vi "BCU诊断标定.vi"(8 "CAN端口":u16(ring), 9 "设备索引号":u16(ring), 10 "CAN卡类型":u32(ring)=21, 11 "Myindex":dbl=1.0) -> (3 "成功":bool)   [LabVIEW 2013] (continued)
                    n2819 = Enqueue Element(queue=w3690, element="强制均衡" ("元素"), error in (no error)=w3689) -> (queue out=w3687:refnum<queue>, error out=w3686:errorcluster)  [unwired: 2 out]
                  }
                }
                n2820 = call <vilib>:"Set Busy.vi"("disable click? (T)"=TRUE) -> ()  [unwired: 3 in, 8 out]
              }
            }
          }
        }
        n2821 = Unbundle By Name(w901) -> ("status"=w900:bool)
        n2822 = Or(x=w900, y=w902) -> (x .or. y?=w903:bool)
      }
      n2823 = Release Queue(queue=w896, force destroy? (F)=TRUE ("强制销毁？(F)"), error in (no error)=w895) -> (error out=w893:errorcluster)  [unwired: 2 out]
      n2824 = call <vilib>:"Clear Errors.vi"("error in (no error)"=w893) -> ()  [unwired: 7 out]
    }
    frame Disabled {
    }
  }
  n2825 = while {
    tunnel: w39 -> [w3702]
    tunnel: w38 -> [w3701]
    tunnel: [w3700] -> w42
    tunnel: [w3699] -> w41
    tunnel: w34 -> [_]
    tunnel: w37 -> [w3691]
    stop <- w3698 stop-if-true
    n2826 = local read "停止"() -> (w3698:bool)
    n2827 = local read "设备索引号"() -> (w3695:u16)
    n2828 = local read "CAN卡类型"() -> (w3696:u32)
    n2829 = local read "CAN端口"() -> (w3694:u16)
    n2830 = call "receiver-8.6.vi"("错误输入（无错误）"=w3691, "CAN端口"=w3694, "设备索引号"=w3695, "CAN卡类型"=w3696) -> ("错误输出"=w3697:errorcluster, "输出簇"=w3693:T25, "接收成功"=w3692:bool)  [unwired: 3 out]
    n2831 = call <vilib>:"Clear Errors.vi"("error in (no error)"=w3697) -> ()  [unwired: 6 in, 1 out]
    n2832 = case shown="真" w3692 {
      tunnel: w3701 -> [w3703 w3709]
      tunnel: w3693 -> [_ w3708]
      tunnel: w3702 -> [w3704 w3707]
      tunnel: [w3704 w3706] -> w3700
      tunnel: [w3703 w3705] -> w3699
      frame False {
      }
      frame True {
        n2833 = Enqueue Element(queue=w3707, element=w3708, error in (no error)=w3709) -> (queue out=w3706:refnum<queue>, error out=w3705:errorcluster)  [unwired: 2 out]
      }
    }
  }
  n2834 = while {
    tunnel: w39 -> [w3717]
    tunnel: w38 -> [w3716]
    stop <- w3710 stop-if-true
    n2835 = local read "停止"() -> (w3710:bool)
    n2836 = local read "控制1"() -> (w3712:bool)
    n2837 = Dequeue Element(queue=w3717, timeout in ms (-1)=200 ("超时毫秒(-1)"), error in (no error)=w3716) -> (element=w3715:T3, error out=w3714:errorcluster)  [unwired: 2 out]
    n2838 = case shown="无错误" w3714 {
      tunnel: w3715 -> [w3722 _]
      tunnel: "写?" -> [w3719 _]
      tunnel: w3712 -> [w3718 _]
      frame No Error {
        n2839 = Unbundle(w3722) -> ("return type"=w3721:u32, "pReceive"=w3720:T26)
        n2840 = for {
          N: w3721 -> [_]
          tunnel: w3720 -> [w3726] mode=indexing
          tunnel: w3719 -> [w3724]
          tunnel: w3718 -> [w3723]
          n2841 = Unbundle By Name(w3726) -> ("ID"=w3727:u32)
          n2842 = call "ID解析.vi"("ID"=w3727) -> ("PDU(1)"=w3725:i32)  [unwired: 10 out]
          n2843 = case shown="18" w3725 {
            tunnel: w3726 -> [_ w3737]
            tunnel: w3724 -> [_ w3729]
            tunnel: w3723 -> [_ w3728]
            frame 0, Default {
            }
            frame 24 {
              n2844 = local read "主从选择"() -> (w3730:enum32{"主板", "从板"})
              n2845 = local read "设备索引号"() -> (w3733:u16)
              n2846 = local read "CAN卡类型"() -> (w3732:u32)
              n2847 = local read "CAN端口"() -> (w3734:u16)
              n2848 = disable-structure shown="禁用" {
                disable-tunnel: w3737 -> [w3740 _]
                frame Disabled {
                  n2849 = call "标定授权读取.vi"("VCI_Receive"=w3740) -> ()  [unwired: 1 out]
                }
                frame Enabled {
                }
              }
              n2850 = case shown="\"从板\"" w3730 {
                tunnel: [0 ("FUNC") w3739] -> w3731
                frame "主板", Default {
                }
                frame "从板" {
                  n2851 = local read "从板号"() -> (w3739:u8)
                }
              }
              n2852 = local read "面板选择"() -> (w3736:T7)
              n2853 = case shown="\"读写参数\", 默认" w3736 {
                tunnel: w3729 -> [w3747 _ _ _]
                tunnel: "命令" -> [w3748 w3848 w4103 w4243]
                tunnel: w3730 -> [w3757 _ w4111 w4251]
                tunnel: w3737 -> [_ _ _ _]
                tunnel: w3737 -> [w3753 w3849 w4105 w4245]
                tunnel: w3734 -> [w3752 w3850 w4106 w4246]
                tunnel: w3733 -> [w3751 w3851 w4107 w4247]
                tunnel: w3732 -> [w3750 w3852 w4108 w4248]
                tunnel: w3731 -> [w3749 _ w4104 w4244]
                tunnel: w3728 -> [w3743 _ _ _]
                frame "读写参数", Default {
                  n2854 = control-ref of="流控帧 2"() -> (w3741:refnum<vi>)
                  n2855 = control-ref of="流控帧"() -> (w3742:refnum<vi>)
                  n2856 = local read "命令序号"() -> (w3746:u8)
                  n2857 = call "多帧接收机制(EV05).vi"("can卡类型"=w3750, "设备索引号"=w3751, "CAN端口"=w3752, "VCI_Receive"=w3753, "命令"=w3748, "板号"=w3749, "流控帧"=w3742, "写?"=w3747, "流控帧2"=w3741, "命令序号"=w3746) -> ("错误信号"=w3744:bool, "错误代码"=w3756:i32, "输出数组"=w3755:u8[], "读错误代码"=w3745:u8[], "结束信号"=w3754:bool)  [unwired: 5 out]
                  n2858 = case shown="真" w3747 {
                    tunnel: w3754 -> [w3767 w3830]
                    tunnel: w3756 -> [w3766 w3829]
                    tunnel: w3746 -> [w3765 _]
                    tunnel: w3755 -> [w3764 _]
                    tunnel: w3748 -> [w3763 _]
                    tunnel: w3757 -> [w3761 w3828]
                    tunnel: w3745 -> [w3760 _]
                    tunnel: w3744 -> [w3759 _]
                    tunnel: w3743 -> [w3758 _]
                    frame False {
                      # "读参数"
                      n2859 = And(x=w3758, y=w3767) -> (x .and. y?=w3762:bool)
                      n2860 = case shown="真" w3762 {
                        tunnel: w3766 -> [_ w3778]
                        tunnel: w3765 -> [_ w3777]
                        tunnel: w3764 -> [_ w3776]
                        tunnel: w3763 -> [_ w3775]
                        tunnel: w3761 -> [_ w3771]
                        tunnel: w3760 -> [_ w3769]
                        tunnel: w3759 -> [_ w3770]
                        frame False {
                        }
                        frame True {
                          n2861 = case shown="假" w3770 {
                            tunnel: w3778 -> [w3787 _]
                            tunnel: w3777 -> [w3786 _]
                            tunnel: w3776 -> [w3785 _]
                            tunnel: w3775 -> [w3783 _]
                            tunnel: w3771 -> [w3779 _]
                            tunnel: w3769 -> [_ w3813]
                            frame False {
                              n2862 = case shown="\"主板\", 默认" w3779 {
                                tunnel: [w3788 _] -> w3782
                                tunnel: [_ w3801] -> w3781
                                frame "主板", Default {
                                n2863 = stacked-sequence {
                                tunnel: [_ w3800] -> w3788
                                frame #0 {
                                n2864 = control-ref of="一级故障"() -> (w3794:refnum<vi>)
                                n2865 = control-ref of="一级故障 2"() -> (w3796:refnum<vi>)
                                n2866 = control-ref of="一级故障 3"() -> (w3797:refnum<vi>)
                                n2867 = control-ref of="加热控制参数"() -> (w3798:refnum<vi>)
                                n2868 = control-ref of="充电控制参数"() -> (w3799:refnum<vi>)
                                n2869 = control-ref of="电池信息"() -> (w3792:refnum<vi>)
                                n2870 = control-ref of="项目信息"() -> (w3795:refnum<vi>)
                                n2871 = control-ref of="项目信息2"() -> (w3793:refnum<vi>)
                                n2872 = control-ref of="高压参数"() -> (w3791:refnum<vi>)
                                n2873 = local read "主板数据"() -> (w3790:T4)
                                n2874 = Bundle(cluster=w3790, "项目信息"=w3795, "一级故障 4"=w3793, "一级故障"=w3794, "一级故障 2"=w3796, "一级故障 3"=w3797, "加热控制参数"=w3798, "充电控制参数"=w3799, "高压参数"=w3791, "电池信息"=w3792) -> (w3789:T4)
                                n2875 = local write "主板数据"(w3789) -> ()
                                }
                                frame #1 {
                                n2876 = control-ref of="主板数据"() -> (w3800:refnum<vi>)
                                }
                                }
                                }
                                frame "从板" {
                                n2877 = stacked-sequence {
                                tunnel: [_ w3812] -> w3801
                                frame #0 {
                                n2878 = control-ref of="从板号"() -> (w3806:refnum<vi>)
                                n2879 = control-ref of="项目信息 2"() -> (w3807:refnum<vi>)
                                n2880 = control-ref of="电池组信息"() -> (w3805:refnum<vi>)
                                n2881 = control-ref of="加热控制参数"() -> (w3808:refnum<vi>)
                                n2882 = control-ref of="一级故障(从板)"() -> (w3809:refnum<vi>)
                                n2883 = control-ref of="二级故障(从板)"() -> (w3810:refnum<vi>)
                                n2884 = control-ref of="三级故障(从板)"() -> (w3811:refnum<vi>)
                                n2885 = control-ref of="均衡参数"() -> (w3804:refnum<vi>)
                                n2886 = local read "从板信息"() -> (w3803:T2)
                                n2887 = Bundle(cluster=w3803, "从板号"=w3806, "项目信息 2"=w3807, "加热控制参数"=w3808, "一级故障(从板)"=w3809, "二级故障(从板)"=w3810, "三级故障(从板)"=w3811, "电池组信息(从板)"=w3805, "均衡参数"=w3804) -> (w3802:T2)
                                n2888 = local write "从板信息"(w3802) -> ()
                                }
                                frame #1 {
                                n2889 = control-ref of="从板信息"() -> (w3812:refnum<vi>)
                                }
                                }
                                }
                              }
                              n2890 = control-ref of="结果"() -> (w3784:refnum<vi>)
                              n2891 = control-ref of="从板个数"() -> (w3780:refnum<vi>)
                              n2892 = call "输出数据解析.vi"("主板引用"=w3782, "错误代码"=w3787, "命令序号"=w3786, "输入数组"=w3785, "命令"=w3783, "从板引用"=w3781, "进度引用"=w3784, "板选择"=w3779, "从板个数"=w3780) -> ()  [unwired: 7 in, 4 out]
                            }
                            frame True {
                              n2893 = Index Array(array=w3813, index #1=0 ("索引"), index #2=1 ("索引")) -> (element #1=w3816:u8, element #2=w3817:u8)
                              n2894 = Join Numbers(hi=w3816, lo=w3817) -> ((hi.lo)=w3815:u16)
                              n2895 = Number To Hexadecimal String(2:w3815) -> (0:w3814:string)  [unwired: 1 out]
                              n2896 = control-ref of="结果"() -> (w3822:refnum<vi>)
                              n2897 = Concatenate Strings("0x" ("字符串"), w3814) -> (w3823:string)
                              n2898 = Build Array(w3823) -> (w3824:string[])
                              n2899 = call "表格编辑.vi"("新元素/子数组"=w3824, "活动单元格:单元格背景色"=u32 16740749, "MCListbox引用句柄"=w3822) -> ()  [unwired: 9 out]
                            }
                          }
                          n2900 = global write "EV05全局变量1.vi" "流控帧 2"(FALSE ("流控帧 2")) -> ()
                          n2901 = global write "EV05全局变量1.vi" "输出数组"(i32[] []) -> ()
                          n2902 = local write "控制1"(FALSE ("控制1")) -> ()
                          n2903 = local write "消除"(FALSE ("消除")) -> ()
                        }
                      }
                    }
                    frame True {
                      # "写参数判定"
                      n2904 = And(x="控制1", y=w3830) -> (x .and. y?=w3827:bool)
                      n2905 = case shown="真" w3827 {
                        tunnel: w3829 -> [_ w3838]
                        tunnel: w3828 -> [_ w3835]
                        frame False {
                        }
                        frame True {
                          n2906 = call <vilib>:"Unset Busy.vi"() -> ()  [unwired: 2 in, 10 out]
                          n2907 = case shown="\"从板\"" w3835 {
                            tunnel: [w3839 w3840] -> w3837
                            frame "主板", Default {
                              n2908 = local read "主板选项"() -> (w3839:string)
                            }
                            frame "从板" {
                              n2909 = local read "从板选项"() -> (w3840:string)
                            }
                          }
                          n2910 = control-ref of="结果"() -> (w3836:refnum<vi>)
                          n2911 = call "输入数据判定.vi"("主从选择"=w3835, "主板选项"=w3837, "进度引用"=w3836, "错误代码"=w3838) -> ("读取超时"=→"读取超时":bool)  [unwired: 3 in, 4 out]
                          n2912 = global write "EV05全局变量1.vi" "流控帧 2"(FALSE ("流控帧 2")) -> ()
                          n2913 = local write "控制1"(FALSE ("控制1")) -> ()
                          n2914 = local write "消除"(FALSE ("消除")) -> ()
                        }
                      }
                      n2915 = global write "EV05全局变量1.vi" "输出数组"(i32[] []) -> ()
                    }
                  }
                }
                frame "版本读取" {
                  n2916 = local read "命令序号"() -> (w3841:u8)
                  n2917 = local read "从板板号"() -> (w3844:u8)
                  n2918 = local read "控制1"() -> (w3845:bool)
                  n2919 = call "多帧接收机制(EV05).vi"("can卡类型"=w3852, "设备索引号"=w3851, "CAN端口"=w3850, "VCI_Receive"=w3849, "命令"=w3848, "板号"=w3844, "命令序号"=w3841) -> ("错误信号"=w3842:bool, "输出数组"=w3853:u8[], "读错误代码"=w3843:u8[], "结束信号"=w3847:bool)  [unwired: 3 in, 6 out]
                  n2920 = And(x=w3845, y=w3847) -> (x .and. y?=w3846:bool)
                  n2921 = case shown="真" w3846 {
                    tunnel: w3853 -> [_ w3861]
                    tunnel: w3841 -> [_ w3860]
                    tunnel: w3848 -> [_ w3859]
                    tunnel: w3843 -> [_ w3855]
                    tunnel: w3842 -> [_ w3854]
                    frame False {
                    }
                    frame True {
                      n2922 = case shown="假" w3854 {
                        tunnel: w3861 -> [w3865 _]
                        tunnel: w3860 -> [w3864 _]
                        tunnel: w3859 -> [w3863 _]
                        tunnel: w3855 -> [w3862 w4089]
                        frame False {
                          n2923 = case shown="89" w3863 {
                            tunnel: w3864 -> [_ w3868]
                            tunnel: w3865 -> [_ w3867]
                            tunnel: w3862 -> [_ _]
                            frame 0, Default {
                            }
                            frame 137 {
                              n2924 = case shown="1" w3868 {
                                tunnel: w3867 -> [_ w3896 w3940 w3960 w4087]
                                frame 0, Default {
                                }
                                frame 1 {
                                w3878 = "." ("字符串")
                                n2925 = Array Subset(array=w3896, index=0 ("索引"), length=14 ("长度")) -> (w3909:u8[])
                                n2926 = Index Array(array=w3896, index=14 ("索引")) -> (element=w3899:u8)
                                n2927 = Index Array(array=w3896, index #1=15 ("索引"), index #2=16 ("索引")) -> (element #1=w3905:u8, element #2=w3906:u8)
                                n2928 = Index Array(array=w3896, index #1=17 ("索引"), index #2=18 ("索引")) -> (element #1=w3900:u8, element #2=w3901:u8)
                                n2929 = call "数组去零.vi"("输入"=w3909) -> ("输出"=w3884:dbl[])
                                n2930 = Join Numbers(hi=w3900, lo=w3901) -> ((hi.lo)=w3897:u16)
                                n2931 = Join Numbers(hi=w3905, lo=w3906) -> ((hi.lo)=w3898:u16)
                                n2932 = Number To Decimal String(number=w3899) -> (decimal integer string=w3891:string)  [unwired: 1 out]
                                n2933 = Byte Array To String(unsigned byte array=w3884) -> (string=w3883:string)
                                n2934 = Number To Decimal String(number=w3897) -> (decimal integer string=w3879:string)  [unwired: 1 out]
                                n2935 = Number To Decimal String(number=w3898) -> (decimal integer string=w3890:string)  [unwired: 1 out]
                                n2936 = Array Subset(array=w3896, index=21 ("索引"), length=7 ("长度")) -> (w3893:u8[])
                                n2937 = Concatenate Strings("V" ("字符串"), w3891, w3878, w3890, w3878, w3879) -> (w3888:string)
                                n2938 = call "数组去零.vi"("输入"=w3893) -> ("输出"=w3876:dbl[])
                                n2939 = Byte Array To String(unsigned byte array=w3876) -> (string=w3874:string)
                                n2940 = call <vilib>:"Space Constant.vi"() -> ("String"=w3875:string)
                                n2941 = Equal?(x=w3874, y=w3875) -> (x = y?=w3880:bool)
                                n2942 = Concatenate Strings("-" ("字符串"), w3874) -> (w3881:string)
                                n2943 = Select(t=w3875, s=w3880, f=w3881) -> (s? t:f=w3877:string)
                                n2944 = Concatenate Strings(w3883, "-" ("字符串"), w3888, w3877) -> (w3870:string)
                                n2945 = local read "项目软件版本"() -> (w3872:string[])
                                n2946 = local read "从板板号"() -> (w3869:u8)
                                n2947 = local write "项目软件版本号"(w3870) -> ()
                                n2948 = Replace Array Subset(array=w3872, new element=w3870, index=w3869) -> (w3871:string[])
                                n2949 = control-ref of="结果"() -> (w3887:refnum<vi>)
                                n2950 = local write "项目软件版本"(w3871) -> ()
                                n2951 = Build Array("项目软件版本     读取完成" ("读取结果")) -> (w3885:string[])
                                n2952 = call "表格编辑(版本读取).vi"("新元素/子数组"=w3885, "活动单元格:单元格背景色"=u32 6618880, "MCListbox引用句柄"=w3887) -> ()  [unwired: 9 out]
                                }
                                frame 2 {
                                w3923 = ""
                                w3920 = "." ("字符串")
                                n2953 = Array Subset(array=w3940, index=0 ("索引"), length=14 ("长度")) -> (w3928:u8[])
                                n2954 = Index Array(array=w3940, index=14 ("索引")) -> (element=w3943:u8)
                                n2955 = Index Array(array=w3940, index #1=15 ("索引"), index #2=16 ("索引")) -> (element #1=w3949:u8, element #2=w3950:u8)
                                n2956 = Index Array(array=w3940, index #1=17 ("索引"), index #2=18 ("索引")) -> (element #1=w3944:u8, element #2=w3945:u8)
                                n2957 = Join Numbers(hi=w3944, lo=w3945) -> ((hi.lo)=w3941:u16)
                                n2958 = Join Numbers(hi=w3949, lo=w3950) -> ((hi.lo)=w3942:u16)
                                n2959 = Number To Decimal String(number=w3941) -> (decimal integer string=w3921:string)  [unwired: 1 out]
                                n2960 = call "数组去零.vi"("输入"=w3928) -> ("输出"=w3927:dbl[])
                                n2961 = Number To Decimal String(number=w3943) -> (decimal integer string=w3935:string)  [unwired: 1 out]
                                n2962 = Number To Decimal String(number=w3942) -> (decimal integer string=w3934:string)  [unwired: 1 out]
                                n2963 = Array Subset(array=w3940, index=21 ("索引"), length=7 ("长度")) -> (w3937:u8[])
                                n2964 = Byte Array To String(unsigned byte array=w3927) -> (string=w3922:string)
                                n2965 = call "数组去零.vi"("输入"=w3937) -> ("输出"=w3919:dbl[])
                                n2966 = Concatenate Strings("V" ("字符串"), w3935, w3920, w3934, w3920, w3921) -> (w3932:string)
                                n2967 = Byte Array To String(unsigned byte array=w3919) -> (string=w3917:string)
                                n2968 = Equal?(x=w3923, y=w3917) -> (x = y?=w3924:bool)
                                n2969 = Concatenate Strings("-" ("字符串"), w3917) -> (w3925:string)
                                n2970 = Select(t=w3923, s=w3924, f=w3925) -> (s? t:f=w3918:string)
                                n2971 = Concatenate Strings(w3922, "-" ("字符串"), w3932, w3918) -> (w3913:string)
                                n2972 = local read "平台软件版本"() -> (w3915:string[])
                                n2973 = local read "从板板号"() -> (w3912:u8)
                                n2974 = local write "平台软件版本号"(w3913) -> ()
                                n2975 = Replace Array Subset(array=w3915, new element=w3913, index=w3912) -> (w3914:string[])
                                n2976 = control-ref of="结果"() -> (w3930:refnum<vi>)
                                n2977 = local write "平台软件版本"(w3914) -> ()
                                n2978 = Build Array("平台软件版本     读取完成" ("读取结果")) -> (w3929:string[])
                                n2979 = call "表格编辑(版本读取).vi"("新元素/子数组"=w3929, "活动单元格:单元格背景色"=u32 6618880, "MCListbox引用句柄"=w3930) -> ()  [unwired: 1 in, 8 out]
                                }
                                frame 3 {
                                n2980 = Index Array(array=w3960, index #1=0 ("索引"), index #2=1 ("索引")) -> (element #1=w3956:u8, element #2=w3957:u8)
                                n2981 = Join Numbers(hi=w3956, lo=w3957) -> ((hi.lo)=w3955:u16)
                                n2982 = case shown="99, 默认" w3955 {
                                tunnel: w3960 -> [w3963 _ w3997]
                                tunnel: w3955 -> [_ _ w3975]
                                frame 0 {
                                n2983 = Index Array(array=w3963, index #1=2 ("索引"), index #2=3 ("索引")) -> (element #1=w3967:u8, element #2=w3966:u8)
                                n2984 = Join Numbers(hi=w3967, lo=w3966) -> ((hi.lo)=w3962:u16)
                                n2985 = for {
                                N: w3962 -> [_]
                                tunnel: w3963 -> [w3972]
                                tunnel: [w3968] -> w3961 mode=indexing
                                i -> [w3971]
                                n2986 = Add(x=w3971, y=4) -> (x+y=w3969:i32)
                                n2987 = Index Array(array=w3972, index=w3969) -> (element=w3968:u8)
                                }
                                "MODEL号" <- w3961
                                }
                                frame 99, Default {
                                }
                                frame 1..40 {
                                w3980 = ""
                                w4001 = "." ("字符串")
                                n2988 = Array Subset(array=w3997, index=2 ("索引"), length=14 ("长度")) -> (w3986:u8[])
                                n2989 = Index Array(array=w3997, index=16 ("索引")) -> (element=w4009:u8)
                                n2990 = Index Array(array=w3997, index #1=17 ("索引"), index #2=18 ("索引")) -> (element #1=w4015:u8, element #2=w4016:u8)
                                n2991 = Index Array(array=w3997, index #1=19 ("索引"), index #2=20 ("索引")) -> (element #1=w4010:u8, element #2=w4011:u8)
                                n2992 = Join Numbers(hi=w4010, lo=w4011) -> ((hi.lo)=w4007:u16)
                                n2993 = Join Numbers(hi=w4015, lo=w4016) -> ((hi.lo)=w4008:u16)
                                n2994 = Number To Decimal String(number=w3975) -> (decimal integer string=w3995:string)  [unwired: 1 out]
                                n2995 = Number To Decimal String(number=w4009) -> (decimal integer string=w4003:string)  [unwired: 1 out]
                                n2996 = call "数组去零.vi"("输入"=w3986) -> ("输出"=w3985:dbl[])
                                n2997 = Number To Decimal String(number=w4008) -> (decimal integer string=w4002:string)  [unwired: 1 out]
                                n2998 = Number To Decimal String(number=w4007) -> (decimal integer string=w4000:string)  [unwired: 1 out]
                                n2999 = Byte Array To String(unsigned byte array=w3985) -> (string=w3987:string)
                                n3000 = Concatenate Strings("第" ("读取结果"), w3995, "模块" ("字符串"), "     读取完成" ("读取结果")) -> (w3988:string)
                                n3001 = Concatenate Strings("V" ("字符串"), w4003, w4001, w4002, w4001, w4000) -> (w3998:string)
                                n3002 = control-ref of="结果"() -> (w3991:refnum<vi>)
                                n3003 = Array Subset(array=w3997, index=23 ("索引"), length=7 ("长度")) -> (w3984:u8[])
                                n3004 = call "数组去零.vi"("输入"=w3984) -> ("输出"=w3979:dbl[])
                                n3005 = Byte Array To String(unsigned byte array=w3979) -> (string=w3976:string)
                                n3006 = Build Array(w3988) -> (w3990:string[])
                                n3007 = control-ref of="模块软件版本 2"() -> (w3992:refnum<vi>)
                                n3008 = local read "模块软件版本"() -> (w3993:T1)
                                n3009 = Equal?(x=w3980, y=w3976) -> (x = y?=w3981:bool)
                                n3010 = call "表格编辑(版本读取).vi"("新元素/子数组"=w3990, "活动单元格:单元格背景色"=u32 6618880, "MCListbox引用句柄"=w3991) -> ()  [unwired: 1 in, 8 out]
                                n3011 = Concatenate Strings("-" ("字符串"), w3976) -> (w3982:string)
                                n3012 = Select(t=w3980, s=w3981, f=w3982) -> (s? t:f=w3978:string)
                                n3013 = Concatenate Strings(w3987, "-" ("字符串"), w3998, w3978) -> (w3977:string)
                                n3014 = case shown="30" w3975 {
                                tunnel: [_ "VERSIONM" "BCUMCAL" "BMUMCAL" "BMURMCAL" "BCUCMCAL" "BCUDMCAL" "SCH" "BSW" "CDD" "DATALAYER" "DATAANALYSIS" "SOC" "SOH" "SOF" "INTRES" "INTCAN" "CARCAN" "CHGCANL" "THM" "CHGM" "HVM" "LVM" "BALM" "SAFEM" "RUNMODEM" "RELAY" "DO" "GBCHGDET" "SUPPLYPOWGDET" "SUMVDET" "CURDET" "TEMPERDET" "CELLVDET" "ISODET" "AI" "DI" "SYSCONF" "ECUCONF"] -> w3974
                                frame 0, Default {
                                }
                                frame 1 {
                                }
                                frame 2 {
                                }
                                frame 3 {
                                }
                                frame 4 {
                                }
                                frame 5 {
                                }
                                frame 6 {
                                }
                                frame 7 {
                                }
                                frame 8 {
                                }
                                frame 9 {
                                }
                                frame 10 {
                                }
                                frame 11 {
                                }
                                frame 12 {
                                }
                                frame 13 {
                                }
                                frame 14 {
                                }
                                frame 15 {
                                }
                                frame 16 {
                                }
                                frame 17 {
                                }
                                frame 18 {
                                }
                                frame 19 {
                                }
                                frame 20 {
                                }
                                frame 21 {
                                }
                                frame 22 {
                                }
                                frame 23 {
                                }
                                frame 24 {
                                }
                                frame 25 {
                                }
                                frame 26 {
                                }
                                frame 27 {
                                }
                                frame 28 {
                                }
                                frame 29 {
                                }
                                frame 30 {
                                }
                                frame 31 {
                                }
                                frame 32 {
                                }
                                frame 33 {
                                }
                                frame 34 {
                                }
                                frame 35 {
                                }
                                frame 36 {
                                }
                                frame 37 {
                                }
                                frame 38 {
                                }
                                }
                                n3015 = case shown="\"全部读取\"" w3993 {
                                tunnel: w3977 -> [w4060 w4068]
                                tunnel: w3975 -> [w4064 w4073]
                                tunnel: w3992 -> [w4066 w4074]
                                tunnel: w3974 -> [w4065 w4072]
                                frame "全部读取" {
                                n3016 = Number To Decimal String(number=w4064) -> (decimal integer string=w4063:string)  [unwired: 1 out]
                                n3017 = Concatenate Strings(w4063, "-" ("元素"), w4065) -> (w4061:string)
                                n3018 = Build Array(w4061, w4060) -> (w4059:string[])
                                n3019 = call "表格编辑(模块版本).vi"("新元素/子数组"=w4059, "MCListbox引用句柄"=w4066) -> ()  [unwired: 1 in, 9 out]
                                }
                                frame "BCUMCAL", Default {
                                n3020 = Number To Decimal String(number=w4073) -> (decimal integer string=w4071:string)  [unwired: 1 out]
                                n3021 = Concatenate Strings(w4071, "-" ("元素"), w4072) -> (w4069:string)
                                n3022 = Build Array(w4069, w4068) -> (w4067:string[])
                                n3023 = call "表格编辑(模块版本).vi"("新元素/子数组"=w4067, "MCListbox引用句柄"=w4074) -> ()  [unwired: 1 in, 9 out]
                                }
                                }
                                }
                                }
                                }
                                frame 4 {
                                n3024 = Array Subset(array=w4087, length=12 ("长度")) -> (w4085:u8[])  [unwired: 1 in]
                                n3025 = Byte Array To String(unsigned byte array=w4085) -> (string=w4084:string)
                                n3026 = call <vilib>:"Trim Whitespace.vi"("string"=w4084) -> ("trimmed string"=w4076:string)  [unwired: 1 in]
                                n3027 = local read "从板板号"() -> (w4075:u8)
                                n3028 = local write "硬件版本号"(w4076) -> ()
                                n3029 = local read "硬件版本"() -> (w4077:string[])
                                n3030 = Replace Array Subset(array=w4077, new element=w4076, index=w4075) -> (w4078:string[])
                                n3031 = local write "硬件版本"(w4078) -> ()
                                n3032 = global write "EV05全局变量1.vi" "写入超时"(TRUE ("写入超时")) -> ()
                                n3033 = control-ref of="结果"() -> (w4082:refnum<vi>)
                                n3034 = Build Array("硬件版本     读取完成" ("读取结果")) -> (w4081:string[])
                                n3035 = call "表格编辑(版本读取).vi"("新元素/子数组"=w4081, "活动单元格:单元格背景色"=u32 6618880, "MCListbox引用句柄"=w4082) -> ()  [unwired: 9 out]
                                }
                              }
                              n3036 = global write "EV05全局变量1.vi" "写入超时"(TRUE ("写入超时")) -> ()
                            }
                          }
                        }
                        frame True {
                          n3037 = Index Array(array=w4089, index #1=0 ("索引"), index #2=1 ("索引")) -> (element #1=w4094:u8, element #2=w4095:u8)
                          n3038 = Join Numbers(hi=w4094, lo=w4095) -> ((hi.lo)=w4093:u16)
                          n3039 = Number To Hexadecimal String(2:w4093) -> (0:w4092:string)  [unwired: 1 out]
                          n3040 = control-ref of="结果"() -> (w4091:refnum<vi>)
                          n3041 = Concatenate Strings("0x" ("字符串"), w4092) -> (w4099:string)
                          n3042 = Build Array(w4099) -> (w4090:string[])
                          n3043 = call "表格编辑(版本读取).vi"("新元素/子数组"=w4090, "活动单元格:单元格背景色"=u32 16740749, "MCListbox引用句柄"=w4091) -> ()  [unwired: 9 out]
                        }
                      }
                      n3044 = global write "EV05全局变量1.vi" "流控帧 2"(FALSE ("流控帧 2")) -> ()
                      n3045 = local write "控制1"(FALSE ("控制1")) -> ()
                      n3046 = local write "消除"(FALSE ("消除")) -> ()
                      n3047 = call <vilib>:"Unset Busy.vi"() -> ()  [unwired: 2 in, 10 out]
                    }
                  }
                }
                frame "其它诊断" {
                  n3048 = local read "命令序号"() -> (w4101:u8)
                  n3049 = call "多帧接收机制(EV05).vi"("can卡类型"=w4108, "设备索引号"=w4107, "CAN端口"=w4106, "VCI_Receive"=w4105, "命令"=w4103, "板号"=w4104, "命令序号"=w4101) -> ("错误代码"=w4110:i32, "输出数组"=w4102:u8[], "读错误代码"=w4100:u8[], "结束信号"=w4109:bool)  [unwired: 3 in, 6 out]
                  n3050 = case shown="真" w4109 {
                    tunnel: w4111 -> [_ w4112]
                    tunnel: w4110 -> [_ _]
                    tunnel: w4102 -> [_ w4113]
                    tunnel: w4101 -> [_ w4116]
                    tunnel: w4100 -> [_ w4114]
                    frame False {
                    }
                    frame True {
                      n3051 = Insert Into Array(array=w4114, new element=w4113) -> (w4115:u8[])  [unwired: 1 in]
                      n3052 = case shown="1" w4116 {
                        tunnel: w4115 -> [_ w4125 w4211]
                        tunnel: w4112 -> [_ _ w4206]
                        frame 0, Default {
                        }
                        frame 1 {
                          n3053 = Index Array(array=w4125) -> (element #1=w4124:u8, element #2=w4123:u8, element #3=w4122:u8)  [unwired: 3 in]
                          n3054 = Join Numbers(hi=w4123, lo=w4122) -> ((hi.lo)=w4121:u16)
                          n3055 = case shown="4" w4124 {
                            tunnel: w4125 -> [_ _ _ _ _ _ _ _ _ _]
                            tunnel: w4121 -> [_ w4128 w4136 w4146 w4156 w4166 w4176 w4186 w4196 _]
                            frame 0, Default {
                              n3056 = local write "继电器超时处理"(FALSE ("继电器超时处理")) -> ()
                            }
                            frame 1 {
                              n3057 = Equal To 0?(x=w4128) -> (x = 0?=w4127:bool)
                              n3058 = local write "正级继电器 12"(w4127) -> ()
                              n3059 = case shown="假" w4127 {
                                tunnel: w4128 -> [w4131 _]
                                frame False {
                                n3060 = local read "正级继电器"() -> (w4133:bool)
                                n3061 = Number To Hexadecimal String(2:w4131) -> (0:w4130:string)  [unwired: 1 out]
                                n3062 = local write "继电器超时处理"(TRUE ("继电器超时处理")) -> ()
                                n3063 = Not(x=w4133) -> (.not. x?=w4132:bool)
                                n3064 = Concatenate Strings("继电器操作失败,0x" ("消息"), w4130) -> ()  [unwired: 1 out]
                                n3065 = local write "正级继电器"(w4132) -> ()
                                }
                                frame True {
                                (unwired) "继电器操作成功!\n继电器操作成功!\n继电器操作成功!"
                                }
                              }
                            }
                            frame 2 {
                              n3066 = Equal To 0?(x=w4136) -> (x = 0?=w4135:bool)
                              n3067 = case shown="假" w4135 {
                                tunnel: w4136 -> [w4142 _]
                                tunnel: [w4140 "继电器操作成功!\n继电器操作成功!\n继电器操作成功!"] -> _
                                frame False {
                                n3068 = local read "负级继电器"() -> (w4138:bool)
                                n3069 = Number To Hexadecimal String(2:w4142) -> (0:w4141:string)  [unwired: 1 out]
                                n3070 = local write "继电器超时处理"(TRUE ("继电器超时处理")) -> ()
                                n3071 = Not(x=w4138) -> (.not. x?=w4139:bool)
                                n3072 = Concatenate Strings("继电器操作失败,0x" ("消息"), w4141) -> (w4140:string)
                                n3073 = local write "负级继电器"(w4139) -> ()
                                }
                                frame True {
                                }
                              }
                              n3074 = local write "正级继电器 2"(w4135) -> ()
                            }
                            frame 3 {
                              n3075 = Equal To 0?(x=w4146) -> (x = 0?=w4145:bool)
                              n3076 = case shown="假" w4145 {
                                tunnel: w4146 -> [w4152 _]
                                tunnel: [w4150 "继电器操作成功!\n继电器操作成功!\n继电器操作成功!"] -> _
                                frame False {
                                n3077 = local read "预充电继电器"() -> (w4148:bool)
                                n3078 = Number To Hexadecimal String(2:w4152) -> (0:w4151:string)  [unwired: 1 out]
                                n3079 = local write "继电器超时处理"(TRUE ("继电器超时处理")) -> ()
                                n3080 = Not(x=w4148) -> (.not. x?=w4149:bool)
                                n3081 = Concatenate Strings("继电器操作失败,0x" ("消息"), w4151) -> (w4150:string)
                                n3082 = local write "预充电继电器"(w4149) -> ()
                                }
                                frame True {
                                }
                              }
                              n3083 = local write "正级继电器 3"(w4145) -> ()
                            }
                            frame 4 {
                              n3084 = Equal To 0?(x=w4156) -> (x = 0?=w4155:bool)
                              n3085 = case shown="假" w4155 {
                                tunnel: w4156 -> [w4162 _]
                                tunnel: [w4160 "继电器操作成功!\n继电器操作成功!\n继电器操作成功!"] -> _
                                frame False {
                                n3086 = local read "加热继电器"() -> (w4159:bool)
                                n3087 = Number To Hexadecimal String(2:w4162) -> (0:w4161:string)  [unwired: 1 out]
                                n3088 = local write "继电器超时处理"(TRUE ("继电器超时处理")) -> ()
                                n3089 = Not(x=w4159) -> (.not. x?=w4158:bool)
                                n3090 = Concatenate Strings("继电器操作失败,0x" ("消息"), w4161) -> (w4160:string)
                                n3091 = local write "加热继电器"(w4158) -> ()
                                }
                                frame True {
                                }
                              }
                              n3092 = local write "正级继电器 5"(w4155) -> ()
                            }
                            frame 5 {
                              n3093 = Equal To 0?(x=w4166) -> (x = 0?=w4165:bool)
                              n3094 = case shown="假" w4165 {
                                tunnel: w4166 -> [w4172 _]
                                tunnel: [w4170 "继电器操作成功!\n继电器操作成功!\n继电器操作成功!"] -> _
                                frame False {
                                n3095 = local read "充电继电器"() -> (w4168:bool)
                                n3096 = Number To Hexadecimal String(2:w4172) -> (0:w4171:string)  [unwired: 1 out]
                                n3097 = local write "继电器超时处理"(TRUE ("继电器超时处理")) -> ()
                                n3098 = Not(x=w4168) -> (.not. x?=w4169:bool)
                                n3099 = Concatenate Strings("继电器操作失败,0x" ("消息"), w4171) -> (w4170:string)
                                n3100 = local write "充电继电器"(w4169) -> ()
                                }
                                frame True {
                                }
                              }
                              n3101 = local write "正级继电器 4"(w4165) -> ()
                            }
                            frame 6 {
                              n3102 = Equal To 0?(x=w4176) -> (x = 0?=w4175:bool)
                              n3103 = local write "正级继电器 6"(w4175) -> ()
                              n3104 = case shown="假" w4175 {
                                tunnel: w4176 -> [w4182 _]
                                tunnel: [w4180 "继电器操作成功!\n继电器操作成功!\n继电器操作成功!"] -> _
                                frame False {
                                n3105 = local read "风机继电器"() -> (w4178:bool)
                                n3106 = Number To Hexadecimal String(2:w4182) -> (0:w4181:string)  [unwired: 1 out]
                                n3107 = local write "继电器超时处理"(TRUE ("继电器超时处理")) -> ()
                                n3108 = Not(x=w4178) -> (.not. x?=w4179:bool)
                                n3109 = Concatenate Strings("继电器操作失败,0x" ("消息"), w4181) -> (w4180:string)
                                n3110 = local write "风机继电器"(w4179) -> ()
                                }
                                frame True {
                                }
                              }
                            }
                            frame 7 {
                              n3111 = Equal To 0?(x=w4186) -> (x = 0?=w4185:bool)
                              n3112 = case shown="假" w4185 {
                                tunnel: w4186 -> [w4191 _]
                                tunnel: [w4189 "继电器操作成功!\n继电器操作成功!\n继电器操作成功!"] -> _
                                frame False {
                                n3113 = local read "加热继电器(从)"() -> (w4187:bool)
                                n3114 = Number To Hexadecimal String(2:w4191) -> (0:w4190:string)  [unwired: 1 out]
                                n3115 = Not(x=w4187) -> (.not. x?=w4188:bool)
                                n3116 = Concatenate Strings("继电器操作失败,0x" ("消息"), w4190) -> (w4189:string)
                                n3117 = local write "加热继电器(从)"(w4188) -> ()
                                }
                                frame True {
                                n3118 = local write "继电器超时处理"(TRUE ("继电器超时处理")) -> ()
                                }
                              }
                              n3119 = local write "正级继电器 7"(w4185) -> ()
                            }
                            frame 8 {
                              n3120 = Equal To 0?(x=w4196) -> (x = 0?=w4195:bool)
                              n3121 = case shown="假" w4195 {
                                tunnel: w4196 -> [w4201 _]
                                tunnel: [w4199 "继电器操作成功!\n继电器操作成功!\n继电器操作成功!"] -> _
                                frame False {
                                n3122 = local read "风机继电器(从)"() -> (w4197:bool)
                                n3123 = Number To Hexadecimal String(2:w4201) -> (0:w4200:string)  [unwired: 1 out]
                                n3124 = Not(x=w4197) -> (.not. x?=w4198:bool)
                                n3125 = Concatenate Strings("继电器操作失败,0x" ("消息"), w4200) -> (w4199:string)
                                n3126 = local write "风机继电器(从)"(w4198) -> ()
                                }
                                frame True {
                                n3127 = local write "继电器超时处理"(TRUE ("继电器超时处理")) -> ()
                                }
                              }
                              n3128 = local write "正级继电器 8"(w4195) -> ()
                            }
                            frame 85, 170 {
                              n3129 = local write "继电器超时处理"(TRUE ("继电器超时处理")) -> ()
                            }
                          }
                        }
                        frame 2 {
                          n3130 = Index Array(array=w4211) -> (element #1=w4210:u8, element #2=w4209:u8, element #3=w4208:u8)  [unwired: 3 in]
                          n3131 = Join Numbers(hi=w4209, lo=w4208) -> ((hi.lo)=w4207:u16)
                          n3132 = case shown="2" w4210 {
                            tunnel: w4211 -> [_ _ _]
                            tunnel: w4207 -> [_ w4215 w4229]
                            tunnel: w4206 -> [_ w4214 _]
                            frame 0, Default {
                              n3133 = local write "继电器超时处理"(FALSE ("继电器超时处理")) -> ()
                            }
                            frame 1 {
                              n3134 = Equal To 0?(x=w4215) -> (x = 0?=w4213:bool)
                              n3135 = case shown="假" w4213 {
                                tunnel: w4215 -> [w4221 _]
                                tunnel: [w4219 "DO控制操作成功!\nDO控制操作成功!\nDO控制操作成功!"] -> _
                                tunnel: w4214 -> [w4218 _]
                                frame False {
                                n3136 = case shown="\"主板\", 默认" w4218 {
                                frame "主板", Default {
                                n3137 = local read "DO1"() -> (w4224:bool)
                                n3138 = Not(x=w4224) -> (.not. x?=w4223:bool)
                                n3139 = local write "DO1"(w4223) -> ()
                                }
                                frame "从板" {
                                n3140 = local read "DO1 2"() -> (w4226:bool)
                                n3141 = Not(x=w4226) -> (.not. x?=w4225:bool)
                                n3142 = local write "DO1 2"(w4225) -> ()
                                }
                                }
                                n3143 = Number To Hexadecimal String(2:w4221) -> (0:w4220:string)  [unwired: 1 out]
                                n3144 = Concatenate Strings("DO控制操作失败,0x" ("消息"), w4220) -> (w4219:string)
                                }
                                frame True {
                                }
                              }
                              n3145 = case shown="\"从板\"" w4214 {
                                tunnel: w4213 -> [w4216 w4217]
                                frame "主板", Default {
                                n3146 = local write "正级继电器 9"(w4216) -> ()
                                }
                                frame "从板" {
                                n3147 = local write "正级继电器 11"(w4217) -> ()
                                }
                              }
                            }
                            frame 2 {
                              n3148 = Equal To 0?(x=w4229) -> (x = 0?=w4228:bool)
                              n3149 = case shown="假" w4228 {
                                tunnel: w4229 -> [w4234 _]
                                tunnel: [w4232 "DO控制操作成功!\nDO控制操作成功!\nDO控制操作成功!"] -> _
                                frame False {
                                n3150 = Number To Hexadecimal String(2:w4234) -> (0:w4233:string)  [unwired: 1 out]
                                n3151 = local read "DO2"() -> (w4231:bool)
                                n3152 = Not(x=w4231) -> (.not. x?=w4230:bool)
                                n3153 = Concatenate Strings("DO控制操作失败,0x" ("消息"), w4233) -> (w4232:string)
                                n3154 = local write "DO2"(w4230) -> ()
                                }
                                frame True {
                                }
                              }
                              n3155 = local write "正级继电器 10"(w4228) -> ()
                            }
                          }
                        }
                      }
                      n3156 = local write "消除"(FALSE ("消除")) -> ()
                      n3157 = global write "EV05全局变量1.vi" "流控帧 2"(FALSE ("流控帧 2")) -> ()
                      n3158 = local write "控制1"(FALSE ("控制1")) -> ()
                      "继电器超时处理" <- TRUE ("控制1")
                    }
                  }
                }
                frame "高压板校正" {
                  n3159 = local read "命令序号"() -> (w4241:u8)
                  n3160 = call "多帧接收机制(EV05).vi"("can卡类型"=w4248, "设备索引号"=w4247, "CAN端口"=w4246, "VCI_Receive"=w4245, "命令"=w4243, "板号"=w4244, "命令序号"=w4241) -> ("错误信号"=w4237:bool, "错误代码"=w4250:i32, "输出数组"=w4242:u8[], "读错误代码"=w4240:u8[], "结束信号"=w4249:bool)  [unwired: 3 in, 5 out]
                  n3161 = local read "控制1"() -> (w4238:bool)
                  n3162 = And(x=w4238, y=w4249) -> (x .and. y?=w4239:bool)
                  n3163 = case shown="真" w4239 {
                    tunnel: w4251 -> [_ w4255]
                    tunnel: w4250 -> [_ _]
                    tunnel: w4242 -> [_ w4253]
                    tunnel: w4241 -> [_ w4254]
                    tunnel: w4240 -> [_ w4256]
                    tunnel: w4237 -> [_ w4257]
                    frame False {
                    }
                    frame True {
                      n3164 = case shown="假" w4257 {
                        tunnel: w4256 -> [_ w4467]
                        tunnel: w4255 -> [_ _]
                        tunnel: w4254 -> [w4262 _]
                        tunnel: w4253 -> [w4261 _]
                        frame False {
                          n3165 = case shown="2" w4262 {
                            tunnel: w4261 -> [_ w4267 w4301 w4331 w4358 w4385 w4412 w4439]
                            frame 0, Default {
                            }
                            frame 1 {
                              n3166 = for {
                                N: 10 -> [_]
                                tunnel: w4267 -> [w4284]
                                shift-right: [w4271] -> w4265
                                shift-left: string[] [] -> [w4273]
                                i -> [w4270]
                                w4278 = 8 ("索引")
                                w4282 = 2 ("y")
                                n3167 = Multiply(x=w4270, y=w4282) -> (x*y=w4283:i32)
                                n3168 = Array Subset(array=w4284, index=w4283, length=w4282) -> (w4281:u8[])
                                n3169 = Index Array(array=w4281) -> (element #1=w4280:u8, element #2=w4279:u8)  [unwired: 2 in]
                                n3170 = call "二进制解析-8.6.vi"("索引"=w4278, "数值"=w4280) -> ("低位子数组"=w4277:i32[])  [unwired: 1 in, 2 out]
                                n3171 = call "二进制解析-8.6.vi"("索引"=w4278, "数值"=w4279) -> ("低位子数组"=w4276:i32[])  [unwired: 1 in, 2 out]
                                n3172 = Insert Into Array(array=w4277, new element=w4276) -> (w4275:i32[])  [unwired: 1 in]
                                n3173 = case shown="2" w4270 {
                                tunnel: [6 15 9 4 2 0 2] -> w4269
                                frame 0, Default {
                                }
                                frame 1 {
                                }
                                frame 2 {
                                }
                                frame 3..5 {
                                }
                                frame 8, 9 {
                                }
                                frame 7 {
                                }
                                frame 6 {
                                }
                                }
                                n3174 = Reverse 1D Array(array=w4275) -> (reversed array=w4274:i32[])
                                n3175 = for {
                                N: w4269 -> [_]
                                tunnel: w4274 -> [w4296] mode=indexing
                                tunnel: [w4292] -> w4272 mode=indexing
                                n3176 = Equal To 0?(x=w4296) -> (x = 0?=w4295:bool)
                                n3177 = Select(t="无", s=w4295, f="故障") -> (s? t:f=w4292:string)
                                }
                                n3178 = Insert Into Array(array=w4273, new element=w4272) -> (w4271:string[])  [unwired: 1 in]
                              }
                              n3179 = call "详细故障分解.vi"("名称"=string[] ["上电自检异常(CellV)", "通讯异常(CellV)", "不更新(CellV)", "未校准(CellV)", "保留", "采样线路断路(CellV)", "18b20上电自检异常(T) ", "18b20通讯异常(T)", "18b20传感器丢失(T)", "18b20传感器无号(T)", "18b20温度异常跳变(T)", "18b20信号线对电源短路(T)", "18b20信号线对地短路(T)", "18b20 CRC校验异常(T)", "NTC上电自检异常(T)", "NTC通讯异常(T)", "NTC传感器丢失(T)", "NTC温度异常跳变(T)", "NTC信号线断路(T)", "NTC信号线对电源短(T)", "NTC信号线对地短路(T)", "上电自检异常(Curr)", "参数异常(Curr)", "不更新(Curr)", "未校准(Curr)", "采样线断开(Curr)", "电流零漂异常(Curr)", "传感器反接(Curr)", "读取实时电流故障(Curr)", "平均电流故障(Curr)", "自检异常(iso)", "前端检测电阻损坏(iso)", "不更新(iso)", "未校准(iso)", "上电自检异常(Sumv_in)", "通讯异常(Sumv_in)", "不更新(Sumv_in)", "未校准(Sumv_in)", "上电自检异常(Sumv_out)", "通讯异常(Sumv_out)", "不更新(Sumv_out)", "未校准(Sumv_out)", "系统时钟自检异常(Clock)", "系统时钟未校准(Clock)", "充电均衡模块不能开启", "充电均衡模块不能关闭", "放电均衡模块不能开启", "放电均衡模块不能关闭"], "故障输入口"=w4265) -> ("输出数组"=w4263:string[][])  [unwired: 1 in, 2 out]
                              n3180 = local write "电池故障"(w4263) -> ()
                            }
                            frame 2 {
                              n3181 = for {
                                N: 5 -> [_]
                                tunnel: w4301 -> [w4318]
                                shift-right: [w4305] -> w4299
                                shift-left: string[] [] -> [w4307]
                                i -> [w4303]
                                w4312 = 8 ("索引")
                                w4316 = 2 ("y")
                                n3182 = Multiply(x=w4303, y=w4316) -> (x*y=w4317:i32)
                                n3183 = Array Subset(array=w4318, index=w4317, length=w4316) -> (w4315:u8[])
                                n3184 = Index Array(array=w4315) -> (element #1=w4314:u8, element #2=w4313:u8)  [unwired: 2 in]
                                n3185 = call "二进制解析-8.6.vi"("索引"=w4312, "数值"=w4314) -> ("低位子数组"=w4311:i32[])  [unwired: 1 in, 2 out]
